vi "ReadMultiLine.vi"(8 "error in (no error)":errorcluster, 10 "Lines to Read/Output":T1={"Total Lines to Read"=2, "Lines to Output"=1}, 11 "refnum in":refnum<file>) -> (0 "error out":errorcluster, 2 "Strings":string, 3 "refnum out":refnum<file>)   [LabVIEW 2014, in "CustomVI.lvlib"]
uses:
  LabView/CustomVI/CustomVI.lvlib
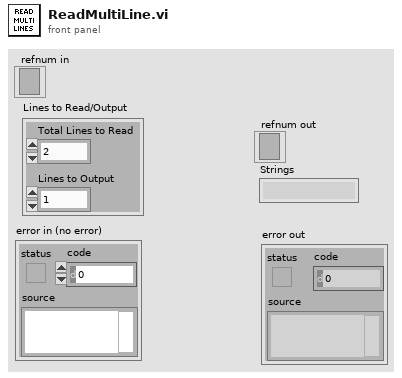
[diagram p1: front panel]
types:
  T1 = cluster{"Total Lines to Read":i32, "Lines to Output":i32}
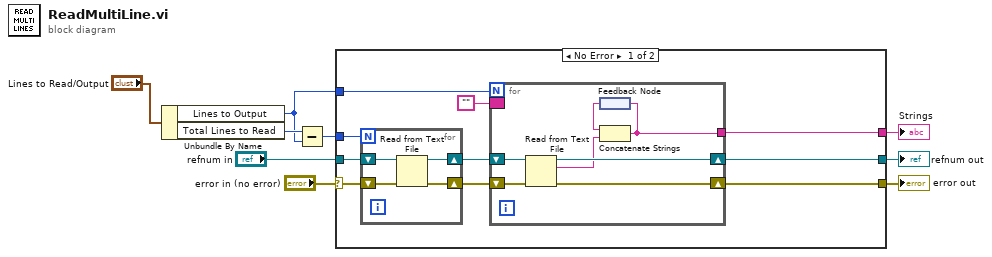
[diagram p0: block diagram]
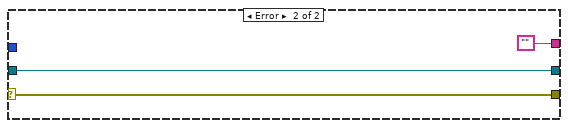
[diagram p2: hidden frame]
diagram:
  n1 = Unbundle By Name("Lines to Read/Output") -> ("Lines to Output"=w1:i32, "Total Lines to Read"=w2:i32)
  n2 = Subtract(x=w2, y=w1) -> (x-y=w7:i32)
  n3 = case shown="No Error" "error in (no error)" {
    selector: "error in (no error)" -> [w16 w33]
    tunnel: [w19 w33] -> w9
    tunnel: w1 -> [w18 _]
    tunnel: w7 -> [w15 _]
    tunnel: "refnum in" -> [w13 w32]
    tunnel: [w12 w32] -> w5
    tunnel: [w10 ""] -> w4
    frame No Error {
      n4 = for {
        N: w15 -> [_]
        shift-right: [w22] -> w17
        shift-left: w16 -> [w23]
        shift-right: [w21] -> w14
        shift-left: w13 -> [w20]
        n5 = Read from Text File(file (use dialog)=w20, error in=w23) -> (refnum out=w21:refnum<file>, error out=w22:errorcluster)  [unwired: 2 in, 2 out]
      }
      n6 = for {
        N: w18 -> [_]
        shift-right: [w29] -> w19
        shift-left: w17 -> [w30]
        shift-right: [w27] -> w12
        shift-left: w14 -> [w28]
        border: "" -> [_]
        tunnel: [w24] -> w10
        n7 = Read from Text File(file (use dialog)=w28, error in=w30) -> (refnum out=w27:refnum<file>, text=w26:string, error out=w29:errorcluster)  [unwired: 2 in, 1 out]
        n8 = feedback #1() -> (w25:string)
        n9 = Concatenate Strings(w25, w26) -> (w24:string)
        n10 = feedback-in #1(w24) -> ()
      }
    }
    frame Error {
    }
  }
  "error out" <- w9
  "refnum out" <- w5
  "Strings" <- w4
